vi "Initialize Function.vi"(0 "functionbase in":refnum<class "functionbase.lvclass">, 11 "error in (no error)":errorcluster) -> (4 "functionbase out":refnum<class "functionbase.lvclass">, 15 "error out":errorcluster)   [LabVIEW 2019, in "LSL.lvlib" / "functionbase.lvclass"]
uses:
  functionbase.lvclass
  functionbase.lvclass/functionbase.ctl
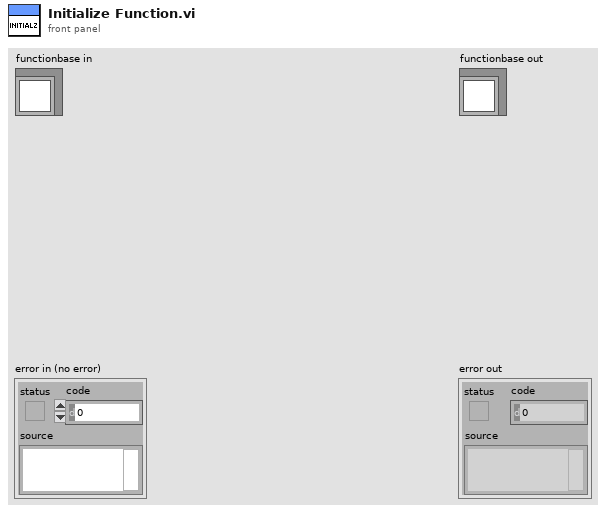
[diagram p1: front panel]
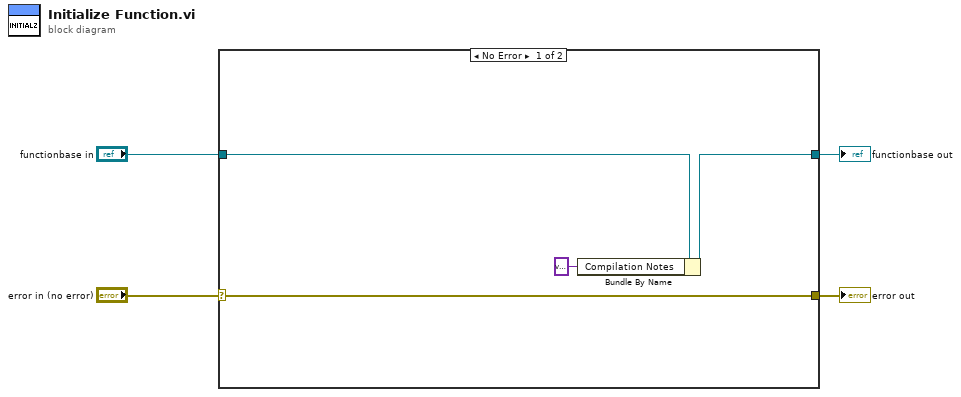
[diagram p0: block diagram]
diagram:
  n1 = case shown="No Error" "error in (no error)" {
    selector: "error in (no error)" -> [w8 w10]
    tunnel: [w8 w10] -> w3
    tunnel: [w5 w9] -> w1
    tunnel: "functionbase in" -> [w6 w9]
    frame No Error {
      n2 = Bundle By Name(cluster=w6, "Compilation Notes"=variant) -> (w5:refnum<class "functionbase.lvclass">)
    }
    frame Error {
    }
  }
  "error out" <- w3
  "functionbase out" <- w1
